vi "TestProto.vi"(8 "error in":errorcluster, 10 "test name":string, 11 "project folder":path) -> (0 "error out":errorcluster, 2 "test result":T1)   [LabVIEW 2019]
uses:
  TestResults.ctl
  <vilib>/gRPC/gRPC Server and Client Template [2]/gRPC Scripting Tools/gRPC Template Creation Utility-release.lvlib
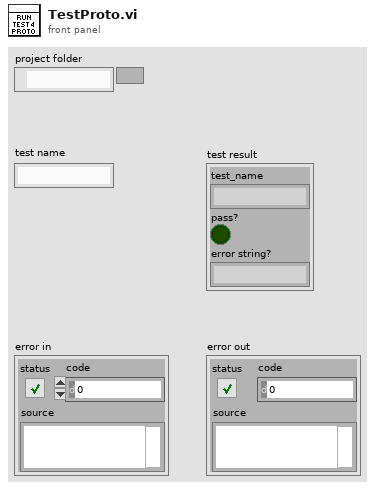
[diagram p1: front panel]
types:
  T1 = typedef "TestResults.ctl" = cluster{"test_name":string, "pass?":bool, "error string?":string}
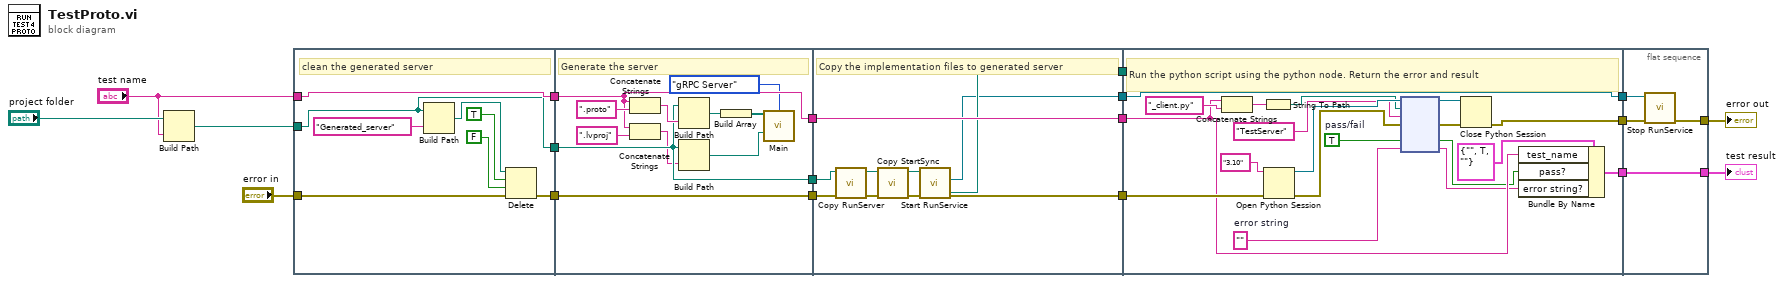
[diagram p0: block diagram]
diagram:
  n1 = Build Path(base path="project folder", name or relative path="test name") -> (appended path=w12:path)
  n2 = flat-sequence {
    tunnel: "error in" -> [w26]
    tunnel: "test name" -> [w27]
    tunnel: w12 -> [w22]
    tunnel: [w22] -> w7
    tunnel: [w27] -> w6
    tunnel: [w25] -> w5
    tunnel: [w33] -> w19
    tunnel: [w36] -> w18
    tunnel: [w35] -> w9
    tunnel: w7 -> [w33]
    tunnel: w6 -> [w36]
    tunnel: w5 -> [w35]
    tunnel: w19 -> [w47]
    tunnel: w18 -> [w48]
    tunnel: [w48] -> w17
    tunnel: [w42] -> w16
    tunnel: [w40] -> w15
    tunnel: w9 -> [w44]
    tunnel: [w39] -> w4
    tunnel: w17 -> [w53]
    tunnel: w16 -> [w66]
    tunnel: w15 -> [_]
    tunnel: w4 -> [w49]
    tunnel: [w56] -> w3
    tunnel: [w50] -> w2
    tunnel: [w49] -> w1
    tunnel: [w70] -> w8
    tunnel: [w69] -> w14
    tunnel: w3 -> [w71]
    tunnel: w2 -> [w70]
    tunnel: w1 -> [w68]
    frame #0 {
      # "clean the generated server"
      n3 = Build Path(base path=w22, name or relative path="Generated_server") -> (appended path=w20:path)
      n4 = Delete(path (use dialog)=w20, entire hierarchy (F)=TRUE, confirm (F)=FALSE, error in=w26) -> (error out=w25:errorcluster)  [unwired: 1 in, 2 out]
    }
    frame #1 {
      # "Generate the server"
      n5 = Concatenate Strings(w36, ".proto" ("string")) -> (w34:string)
      n6 = Concatenate Strings(w36, ".lvproj" ("string")) -> (w29:string)
      n7 = Build Path(base path=w33, name or relative path=w34) -> (appended path=w31:path)
      n8 = Build Path(base path=w33, name or relative path=w29) -> (appended path=w30:path)
      n9 = Build Array(w31) -> (w38:path[])
      n10 = call <vilib>:"Main.vi"("Proto File Path"=w38, "Generate"=enum16{"gRPC Server", "gRPC Client", "Both"}."gRPC Server", "Target Project"=w30) -> ()  [unwired: 13 in]
    }
    frame #2 {
      # "Copy the implementation files to generated server"
      n11 = call "Copy RunServer.vi"("error in (no error)"=w44, "project folder"=w47) -> ("error out"=w45:errorcluster, "project folder out"=w46:path)  [unwired: 8 in]
      n12 = call "Copy StartSync.vi"("error in (no error)"=w45, "project folder"=w46) -> ("error out"=w43:errorcluster, "project folder out"=w41:path)  [unwired: 8 in]
      n13 = call "Start RunService.vi"("error in (no error)"=w43, "project folder"=w41) -> ("error out"=w42:errorcluster, "vi reference"=w39:refnum<vi>, "project folder out"=w40:path)  [unwired: 7 in]
    }
    frame #3 {
      w58 = ""  # error string
      w59 = TRUE  # pass/fail
      # "Run the python script using the python node. Return the error and result"
      n14 = Concatenate Strings(w53, "_client.py" ("string")) -> (w62:string)
      n15 = String To Path(string=w62) -> (path=w61:path)
      n16 = Open Python Session(python version="3.10" ("Python version"), 3:w66) -> (session out=w64:refnum<k35>, error out=w63:errorcluster)  [unwired: 1 in]
      n17 = node(w64, w61, "TestServer" ("function name"), w63, w59, w58) -> (w55:refnum<k35>, w57:errorcluster, w52:bool, w51:string)  [unwired: 2 in, 2 out]
      n18 = Close Python Session(session in=w55, error in=w57) -> (11:w56:errorcluster)
      n19 = Bundle By Name(cluster=T1 {"test_name"="", "pass?"=TRUE, "error string?"=""} ("input cluster"), "test_name"=w53, "pass?"=w52, "error string?"=w51) -> (w50:T1)
    }
    frame #4 {
      n20 = call "Stop RunService.vi"("error in (no error)"=w71, "vi reference"=w68) -> ("error out"=w69:errorcluster)  [unwired: 9 in]
    }
  }
  "error out" <- w14
  "test result" <- w8
